vi "CMN_toTPNT.vi"(5 "timeout":i32=3000, 7 "error in (no error)":errorcluster, 8 "respond to":string, 9 "command":string) -> (0 "error out":errorcluster, 2 "reply":string)   [LabVIEW 2016]
doc: "Sends commands to the module manager"
panel:
  in  "TPNT_CmdStruct":cluster{"command":string, "respondTo":string}
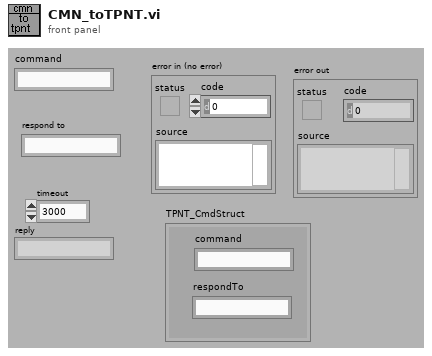
[diagram p1: front panel]
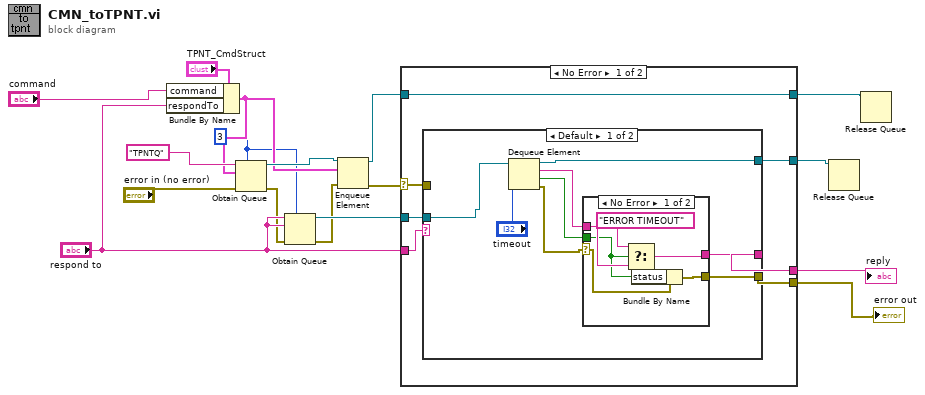
[diagram p0: block diagram]
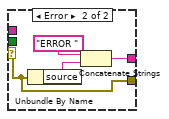
[diagram p2: hidden frame]
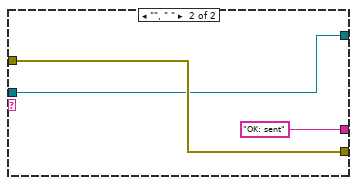
[diagram p3: hidden frame]
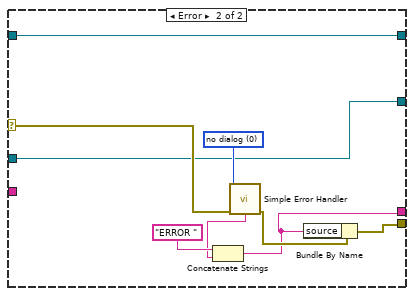
[diagram p4: hidden frame]
diagram:
  w1 = 3 ("max queue size (-1, unlimited)")
  n1 = Bundle By Name(cluster="TPNT_CmdStruct", "command"="command", "respondTo"="respond to") -> (w10:cluster{"command":string, "respondTo":string})
  n2 = Obtain Queue(max queue size (-1, unlimited)=w1, name (unnamed)="TPNTQ", element data type=w10, error in (no error)="error in (no error)") -> (queue out=w17:refnum<queue>, error out=w4:errorcluster)  [unwired: 1 in, 1 out]
  n3 = Obtain Queue(max queue size (-1, unlimited)=w1, name (unnamed)="respond to", element data type="respond to", error in (no error)=w4) -> (queue out=w5:refnum<queue>, error out=w3:errorcluster)  [unwired: 1 in, 1 out]
  n4 = Enqueue Element(queue=w17, element=w10, error in (no error)=w3) -> (queue out=w8:refnum<queue>, error out=w12:errorcluster)  [unwired: 2 out]
  n5 = case shown="No Error" w12 {
    selector: w12 -> [w21 w54]
    tunnel: [w24 w48] -> w15
    tunnel: [w23 w51] -> w13
    tunnel: "respond to" -> [w22 _]
    tunnel: w8 -> [w20 w47]
    tunnel: [w20 w47] -> w7
    tunnel: w5 -> [w19 w46]
    tunnel: [w18 w46] -> w2
    frame No Error {
      n6 = case shown="Default" w22 {
        tunnel: w21 -> [_ w44]
        tunnel: [w30 "OK: sent"] -> w24
        tunnel: [w27 w44] -> w23
        tunnel: w19 -> [w26 w43]
        tunnel: [w25 w43] -> w18
        frame Default {
          n7 = Dequeue Element(queue=w26, timeout in ms (-1)="timeout") -> (queue out=w25:refnum<queue>, element=w28:string, timed out?=w29:bool, error out=w31:errorcluster)  [unwired: 1 in]
          n8 = case shown="No Error" w31 {
            selector: w31 -> [w34 w39]
            tunnel: [w36 w40] -> w30
            tunnel: w29 -> [w35 _]
            tunnel: w28 -> [w37 _]
            tunnel: [w33 w39] -> w27
            frame No Error {
              n9 = Select(t="ERROR TIMEOUT", s=w35, f=w37) -> (s? t:f=w36:string)
              n10 = Bundle By Name(cluster=w34, "status"=w35) -> (w33:errorcluster)
            }
            frame Error {
              n11 = Unbundle By Name(w39) -> ("source"=w41:string)
              n12 = Concatenate Strings("ERROR ", w41) -> (w40:string)
            }
          }
        }
        frame "", " " {
        }
      }
    }
    frame Error {
      w53 = u16 0 items=["no dialog", "OK message", "continue or stop message"] ("type of dialog (OK msg:1)")
      n13 = call <vilib>:"Simple Error Handler.vi"("type of dialog (OK msg:1)"=w53, "error in (no error)"=w54) -> ("error out"=w52:errorcluster, "message"=w49:string)  [unwired: 6 out]
      n14 = Concatenate Strings("ERROR ", w49) -> (w48:string)
      n15 = Bundle By Name(cluster=w52, "source"=w48) -> (w51:errorcluster)
    }
  }
  "reply" <- w15
  "error out" <- w13
  n16 = Release Queue(queue=w2) -> ()  [unwired: 1 in, 4 out]
  n17 = Release Queue(queue=w7) -> ()  [unwired: 1 in, 4 out]
